vi "Flush Serial Buffer.vi"(8 "error in (no error)":errorcluster, 11 "VISA resource name in":refnum<visa-resource-name>) -> (0 "error out":errorcluster, 3 "VISA resource name out":refnum<visa-resource-name>)   [LabVIEW 2015]
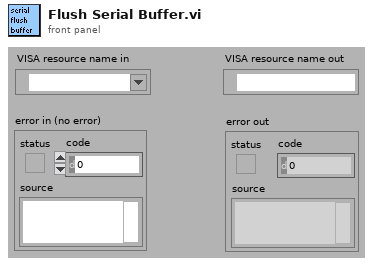
[diagram p1: front panel]
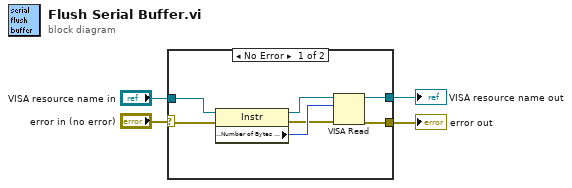
[diagram p0: block diagram]
diagram:
  n1 = case shown="No Error" "error in (no error)" {
    selector: "error in (no error)" -> [w9 w13]
    tunnel: "VISA resource name in" -> [w8 w12]
    tunnel: [w6 w13] -> w2
    tunnel: [w5 w12] -> w1
    frame No Error {
      n2 = property class="Instr"(reference=w8, error in=w9) -> (reference out=w11:refnum<visa-resource-name>, error out=w7:errorcluster, "Serial Settings:Number of Bytes at Serial Port"=w10:u32)
      n3 = VISA Read(VISA resource name=w11, byte count=w10, error in (no error)=w7) -> (VISA resource name out=w5:refnum<visa-resource-name>, error out=w6:errorcluster)  [unwired: 2 out]
    }
    frame Error {
    }
  }
  "error out" <- w2
  "VISA resource name out" <- w1
